vi "convert_string_to_int32Array.vi"(2 "Max Elements Count (All)":i32=-1, 3 "default (0)":i32, 4 "string in":string) -> (0 "int32 array size out":i32 caption="int32 array size", 1 "int32 array out":i32[](array[numeric]))   [LabVIEW 2014, in "rszvl_rsidr_core.lvlib"]
uses:
  rszvl_rsidr_core.lvlib
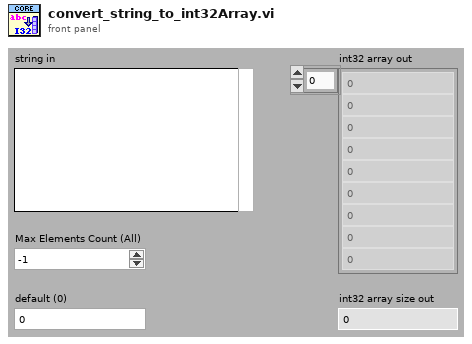
[diagram p1: front panel]
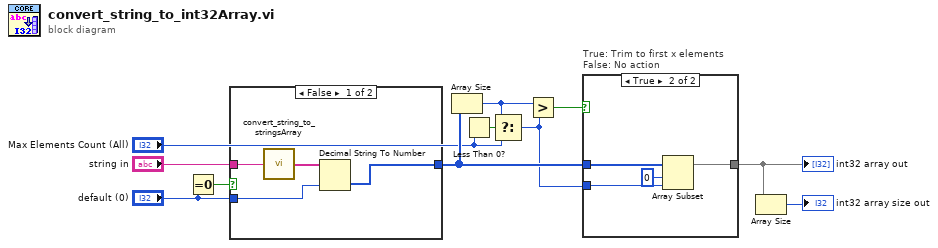
[diagram p0: block diagram]
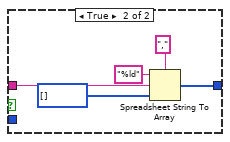
[diagram p3: hidden frame]
diagram:
  n1 = Equal To 0?(x="default (0)") -> (x = 0?=w8:bool)
  n2 = case shown="False" w8 {
    tunnel: "string in" -> [w15 w17]
    tunnel: [w13 w16] -> w4
    tunnel: "default (0)" -> [w12 _]
    frame False {
      n3 = call "convert_string_to_stringsArray.vi"("String in"=w15) -> ("string array out"=w14:string[])  [unwired: 3 in, 1 out]
      n4 = Decimal String To Number(string=w14, default (0L)=w12) -> (number=w13:i32[])  [unwired: 1 in, 1 out]
    }
    frame True {
      n5 = Spreadsheet String To Array(delimiter (Tab)=",", format string="%ld", spreadsheet string=w17, array type (2D Dbl)=i32[] [] ("List Power Results")) -> (array=w16:i32[])
    }
  }
  n6 = Array Size(array=w4) -> (size(s)=w6:i32)
  n7 = Less Than 0?(x="Max Elements Count (All)") -> (x < 0?=w7:bool)
  n8 = Select(t=w6, s=w7, f="Max Elements Count (All)") -> (s? t:f=w2:i32)
  n9 = Greater?(x=w6, y=w2) -> (0:w5:bool)
  n10 = case "True: Trim to first x elements\nFalse: No action" shown="True" w5 {
    tunnel: [w21 w22] -> w1
    tunnel: w4 -> [w21 w25]
    tunnel: w2 -> [_ w23]
    frame False {
    }
    frame True {
      n11 = Array Subset(array=w25, index=0, length=w23) -> (w22:i32[])
    }
  }
  "int32 array out" <- w1
  n12 = Array Size(array=w1) -> (size(s)=→"int32 array size out":i32)
